vi "Packet Get n Bytes.vi"(8 "error in (no error)":errorcluster, 9 "n":i32, 10 "Data":u8[](array[numeric]), 11 "Packet in":refnum<class "Packet.lvclass">) -> (0 "error out":errorcluster, 2 "Data out":u8[](array[numeric]), 3 "Packet out":refnum<class "Packet.lvclass">)   [LabVIEW 2019, in "Packet.lvclass"]
uses:
  Packet.lvclass
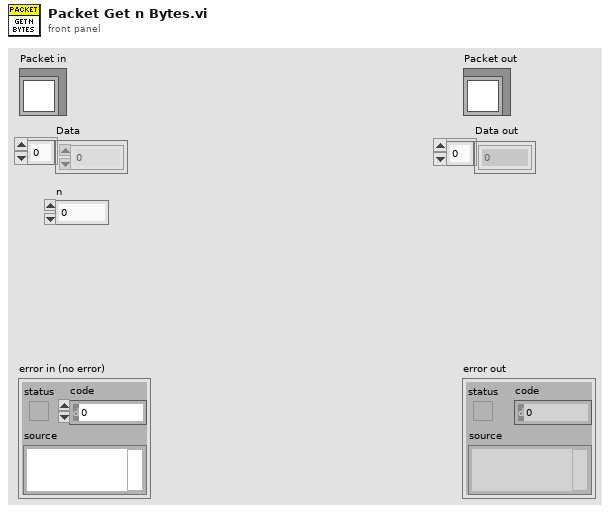
[diagram p1: front panel]
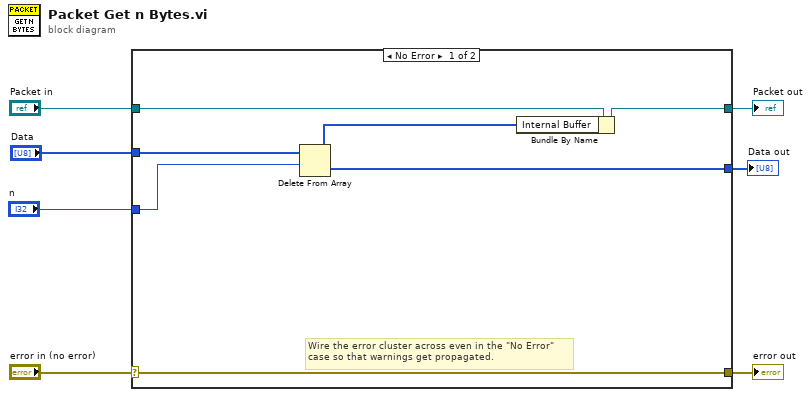
[diagram p0: block diagram]
diagram:
  n1 = case shown="No Error" "error in (no error)" {
    selector: "error in (no error)" -> [w13 w16]
    tunnel: [w13 w16] -> w6
    tunnel: [w12 w15] -> w4
    tunnel: "Packet in" -> [w14 w15]
    tunnel: "Data" -> [w11 _]
    tunnel: "n" -> [w10 _]
    tunnel: [w8 _] -> w1
    frame No Error {
      # "Wire the error cluster across even in the \"No Error\"\ncase so that warnings get propagated."
      n2 = Delete From Array(array=w11, length=w10) -> (deleted portion=w8:u8[], array with subset deleted=w9:u8[])  [unwired: 1 in]
      n3 = Bundle By Name(cluster=w14, "Internal Buffer"=w9) -> (w12:refnum<class "Packet.lvclass">)
    }
    frame Error {
    }
  }
  "error out" <- w6
  "Packet out" <- w4
  "Data out" <- w1
